vi "test variant to json time.vi"(8 "error in (no error)":errorcluster) -> (0 "error out":errorcluster)   [LabVIEW 2019, in "labview_json_tests.lvlib"]
uses:
  labview_json_tests.lvlib
  lib/labview_json.lvlib
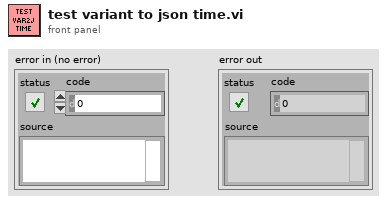
[diagram p1: front panel]
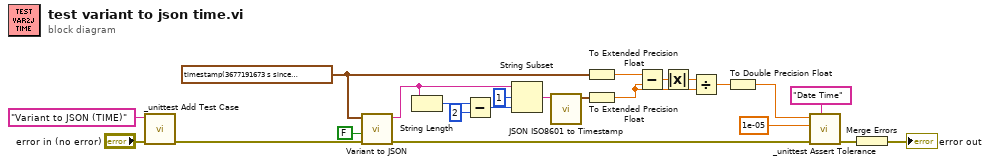
[diagram p0: block diagram]
diagram:
  w12 = timestamp(3677191673.3029866 s since 1904-01-01) ("Time Stamp")
  n1 = call "_unittest Add Test Case.vi"("error in (no error)"="error in (no error)", "Test Case"="Variant to JSON (TIME)") -> ("error out"=w20:errorcluster)  [unwired: 9 in]
  n2 = call "Variant to JSON.vi"("error in (no error)"=w20, "Pretty Print? (F)"=FALSE, "Variant in"=w12) -> ("error out"=w7:errorcluster, "JSON"=w17:string)  [unwired: 7 in]
  n3 = String Length(string=w17) -> (length=w16:i32)
  n4 = Subtract(x=w16, y=2) -> (x-y=w14:i32)
  n5 = String Subset(string=w17, offset (0)=1, length (rest)=w14) -> (substring=w19:string)
  n6 = call "JSON ISO8601 to Timestamp.vi"("ISO 8601 Date Time"=w19) -> ("Local Time Stamp"=w13:timestamp)  [unwired: 10 in]
  n7 = To Extended Precision Float(1:w12) -> (0:w9:ext)
  n8 = To Extended Precision Float(1:w13) -> (0:w8:ext)
  n9 = Subtract(x=w9, y=w8) -> (x-y=w11:ext)
  n10 = Absolute Value(x=w11) -> (abs(x)=w10:ext)
  n11 = Divide(x=w10, y=w8) -> (x/y=w5:ext)
  n12 = To Double Precision Float(number=w5) -> (double precision float=w2:dbl)
  n13 = call "_unittest Assert Tolerance.vi"("Message"="Date Time", "error in (no error)"=w7, "Tollerance (1E-5)"=1e-05, "Actual Value"=w2) -> ("error out"=w6:errorcluster)  [unwired: 7 in]
  n14 = Merge Errors(w6) -> (→"error out":errorcluster)
